vi "connect Channel.vi"(8 "error in (no error)":errorcluster, 10 "Channel Name":string, 11 "2575 in":refnum<class "2575.lvclass">) -> (0 "error out":errorcluster, 3 "2575 out":refnum<class "2575.lvclass">)   [LabVIEW 2019, in "2575.lvlib" / "2575.lvclass"]
uses:
  Library/2575.lvclass
  C:/Users/rdexter/Desktop/Built/SwitchMatrix.lvlibp/SwitchMatrix.lvclass
  Library/2575.lvclass/2575.ctl
  builds/Instruments/SwitchMatrix.lvlibp/Accessors/Read Relay Name.vi
  <instrlib>/niSwitch/niSwitch.llb/niSwitch Connect Channels (Single).vi
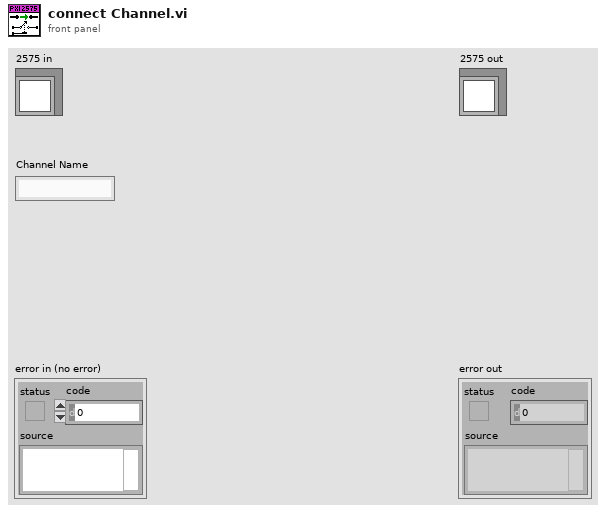
[diagram p1: front panel]
types:
  T1 = typedef "2575.lvlib/2575.lvclass/Device Channel Name.ctl" = string[]
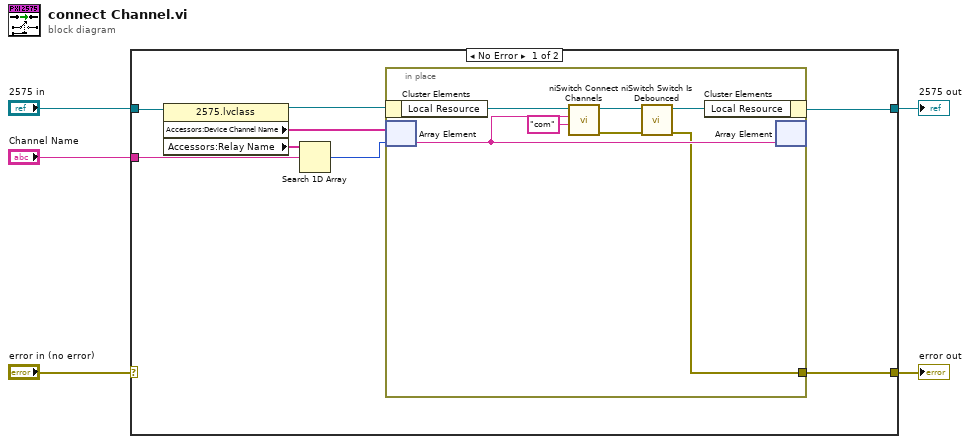
[diagram p0: block diagram]
diagram:
  n1 = case shown="No Error" "error in (no error)" {
    selector: "error in (no error)" -> [_ w22]
    tunnel: [w6 w22] -> w4
    tunnel: [w13 w21] -> w2
    tunnel: "2575 in" -> [w12 w21]
    tunnel: "Channel Name" -> [w9 _]
    frame No Error {
      n2 = property class="2575.lvclass"(reference=w12) -> (reference out=w11:refnum<class "2575.lvclass">, "Accessors:Device Channel Name"=w8:T1, "Accessors:Relay Name"=w10:string[])  [unwired: 1 in, 1 out]
      n3 = Search 1D Array(1D array=w10, element=w9) -> (index of element=w7:i32)  [unwired: 1 in]
      n4 = in-place {
        in-place-border: [w14] -> w6
        n5 = in-place-cluster #1(w11) -> ("Local Resource"=w20:refnum<k15>)
        n6 = in-place-array #2(w8, w7) -> (w15:string)
        n7 = call-poly <instrlib>:"niSwitch Connect Channels.vi"("channel 2"="com", "channel 1"=w15, "instrument handle"=w20) -> ("error out"=w17:errorcluster, "instrument handle out"=w19:refnum<k15>)  [unwired: 7 in]
        n8 = call <instrlib>:"niSwitch Switch Is Debounced.vi"("error in (no error)"=w17, "instrument handle"=w19) -> ("error out"=w14:errorcluster, "instrument handle out"=w18:refnum<k15>)  [unwired: 7 in, 1 out]
        n9 = in-place-cluster #1("Local Resource"=w18) -> (w13:refnum<class "2575.lvclass">)
        n10 = in-place-array #2(w15) -> ()  [unwired: 2 out]
      }
    }
    frame Error {
    }
  }
  "error out" <- w4
  "2575 out" <- w2
